vi "TotalCost_Storage.vi"(11 "Numeric":dbl) -> ()   [LabVIEW 2019]
uses:
  <vilib>/Utility/config.llb/Read Key (Double).vi
  <vilib>/Utility/config.llb/Write Key (Double).vi
  <vilib>/Utility/config.llb/NI_LVConfig.lvlib
panel:
  out "value":dbl
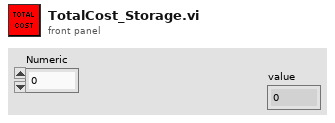
[diagram p1: front panel]
types:
  T1 = typedef "NI_LVConfig.lvlib/Config Data RefNum.ctl" = refnum<k1>
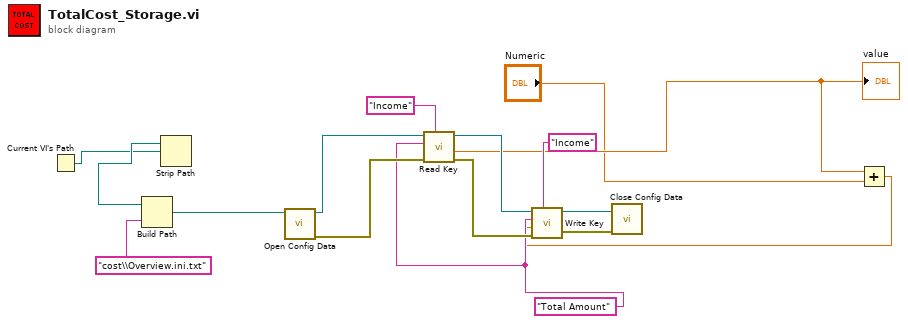
[diagram p0: block diagram]
diagram:
  w4 = "Total Amount" ("key")
  n1 = Current VI's Path() -> (path=w14:path)
  n2 = Strip Path(path=w14) -> (stripped path=w16:path)  [unwired: 1 out]
  n3 = Build Path(base path=w16, name or relative path="cost\\Overview.ini.txt") -> (appended path=w13:path)
  n4 = call <vilib>:"Open Config Data.vi"("configuration file path"=w13) -> ("error out"=w8:errorcluster, "refnum"=w9:T1)  [unwired: 8 in, 1 out]
  n5 = call-poly <vilib>:"Read Key.vi"("section"="Income", "error in (no error)"=w8, "key"=w4, "refnum"=w9) -> ("error out"=w7:errorcluster, "value"=w3:dbl, "refnum out"=w6:T1)  [unwired: 4 in, 1 out]
  "value" <- w3
  n6 = Add(x=w3, y="Numeric") -> (x+y=w1:dbl)
  n7 = call-poly <vilib>:"Write Key.vi"("section"="Income", "error in (no error)"=w7, "value"=w1, "key"=w4, "refnum"=w6) -> ("error out"=w11:errorcluster, "refnum out"=w12:T1)  [unwired: 4 in, 1 out]
  n8 = call <vilib>:"Close Config Data.vi"("error in (no error)"=w11, "refnum"=w12) -> ()  [unwired: 8 in, 2 out]
